vi "RequestIntegerUpdate.vi"(8 "error in (no error)":errorcluster, 10 "NewVal":i32, 11 "Controller in":refnum<class "Controller.lvclass">) -> (0 "error out":errorcluster, 3 "Controller out":refnum<class "Controller.lvclass">)   [LabVIEW 2020, in "Controller.lvclass"]
uses:
  Controller.lvclass
  Controller.lvclass/Controller.ctl
  Model/Model.lvclass
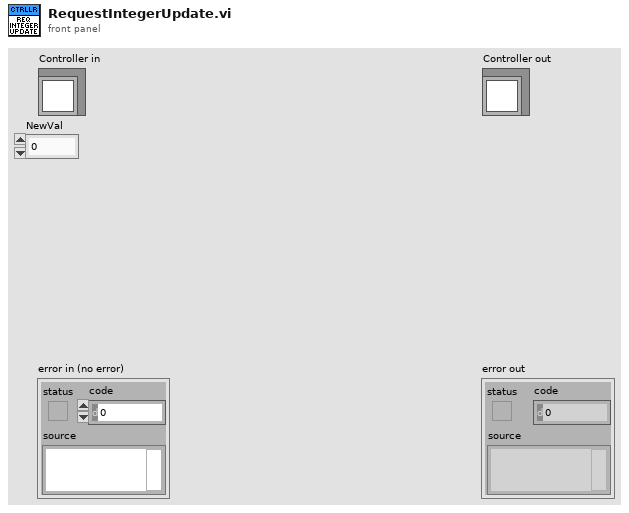
[diagram p1: front panel]
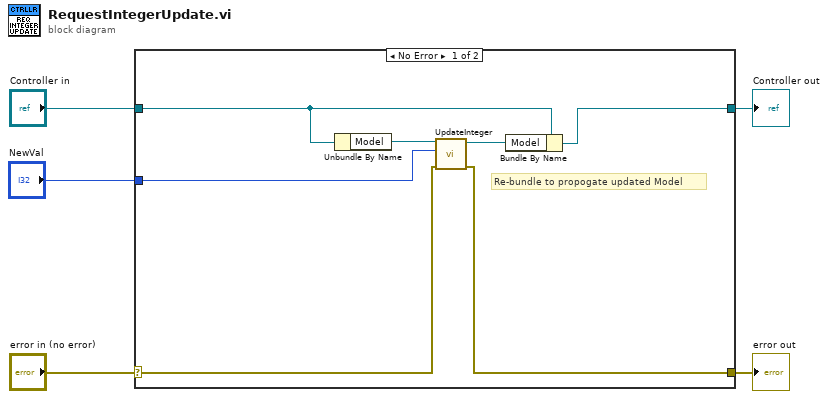
[diagram p0: block diagram]
diagram:
  n1 = case shown="No Error" "error in (no error)" {
    selector: "error in (no error)" -> [w11 w14]
    tunnel: [w6 w14] -> w4
    tunnel: [w7 w13] -> w2
    tunnel: "Controller in" -> [w9 w13]
    tunnel: "NewVal" -> [w10 _]
    frame No Error {
      # "Re-bundle to propogate updated Model"
      n2 = Unbundle By Name(w9) -> ("Model"=w12:refnum<class "Model.lvclass">)
      n3 = call "UpdateInteger.vi"("error in (no error)"=w11, "NewVal"=w10, "Model in"=w12) -> ("error out"=w6:errorcluster, "Model out"=w8:refnum<class "Model.lvclass">)  [unwired: 7 in]
      n4 = Bundle By Name(cluster=w9, "Model"=w8) -> (w7:refnum<class "Controller.lvclass">)
    }
    frame Error {
    }
  }
  "error out" <- w4
  "Controller out" <- w2
